vi "GT Get Sts Ext Mdl.vi"(7 "pStatus":u16, 8 "error in (no error)":errorcluster caption="错误输入（无错误）", 9 "chn":i16, 10 "mdl":i16, 11 "cardNum":i16) -> (0 "error out":errorcluster caption="错误输出", 3 "function return":i16, 5 "pStatus out":u16)   [LabVIEW 2020, in "gts.lvlib"]
doc: "GT_API GT_GetStsExtMdl(short cardNum,short mdl,short chn,unsigned short *pStatus);"
uses:
  gts.lvlib
  dll/32bit/multi_card/gts.dll
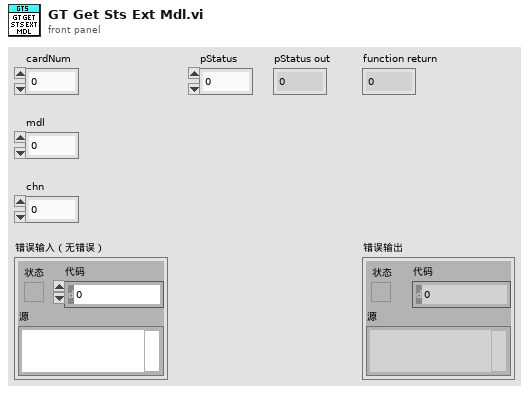
[diagram p1: front panel]
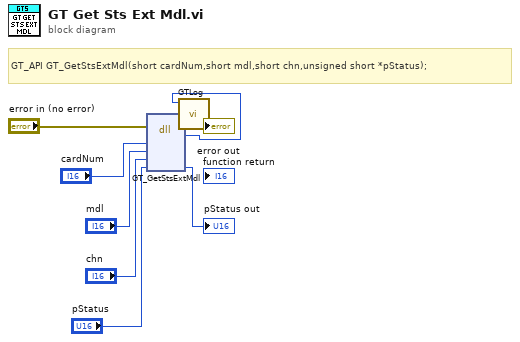
[diagram p0: block diagram]
diagram:
  # "GT_API GT_GetStsExtMdl(short cardNum,short mdl,short chn,unsigned short *pStatus);"
  n1 = dll-call lib="C:/1228/dll/32bit/multi_card/gts.dll" fn="GT_GetStsExtMdl"(error in="error in (no error)", "cardNum"="cardNum", "mdl"="mdl", "chn"="chn", "pStatus"="pStatus") -> (error out=w3:errorcluster, w1:i16, "pStatus"=→"pStatus out":u16)  [unwired: 5 in, 1 out]
  n2 = call "GTLog.vi"("error in (no error)"=w3, "Numeric"=w1) -> ("error out"=→"error out":errorcluster)  [unwired: 9 in]
